vi "init.vi"() -> (0 "error out":errorcluster, 3 "Modules":T1)   [LabVIEW 2025]
uses:
  <vilib>/Utility/sysdir.llb/System Directory Type.ctl
  Libraries/USB IO/USB IO.lvlib
  Libraries/Power Supply/Power Supply.lvlib
  Libraries/Motor/Motor.lvlib
  Libraries/Wheatstone Bridge/Wheatstone Bridge.lvlib
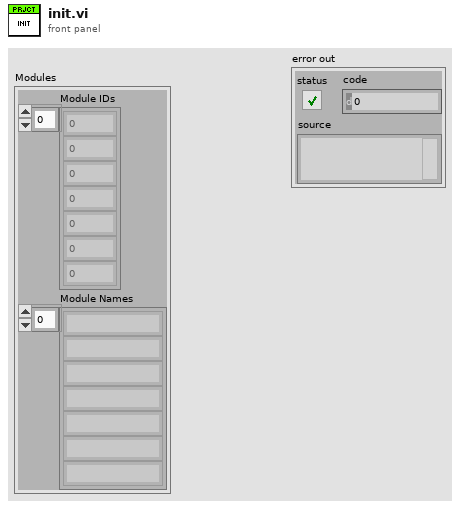
[diagram p1: front panel]
types:
  T1 = cluster{"Module IDs":i32[], "Module Names":string[]}
  T2 = typedef "System Directory Type.ctl" = i32
  T3 = typedef "Hardware Selection.ctl" = enum16{"Simulation", "USB-6000", "USB-6001", "Arduino Uno"}
  T4 = typedef "hardware-selection.ctl" = enum16{"Parent", "Simulation", "PSP-603"}
  T5 = typedef "Motor Selection.ctl" = enum16{"Stepper", "CL57RS"}
  T6 = typedef "Wheatstone Bridge.lvlib/Wheatstone Bridge.lvclass/Hardware Selection.ctl" = enum16{"Wheatstone Bridge", "NI-9237"}
  T7 = cluster{"IO":T3, "Power_supply":T4, "Motor":T5, "Torque Transducer":T6}
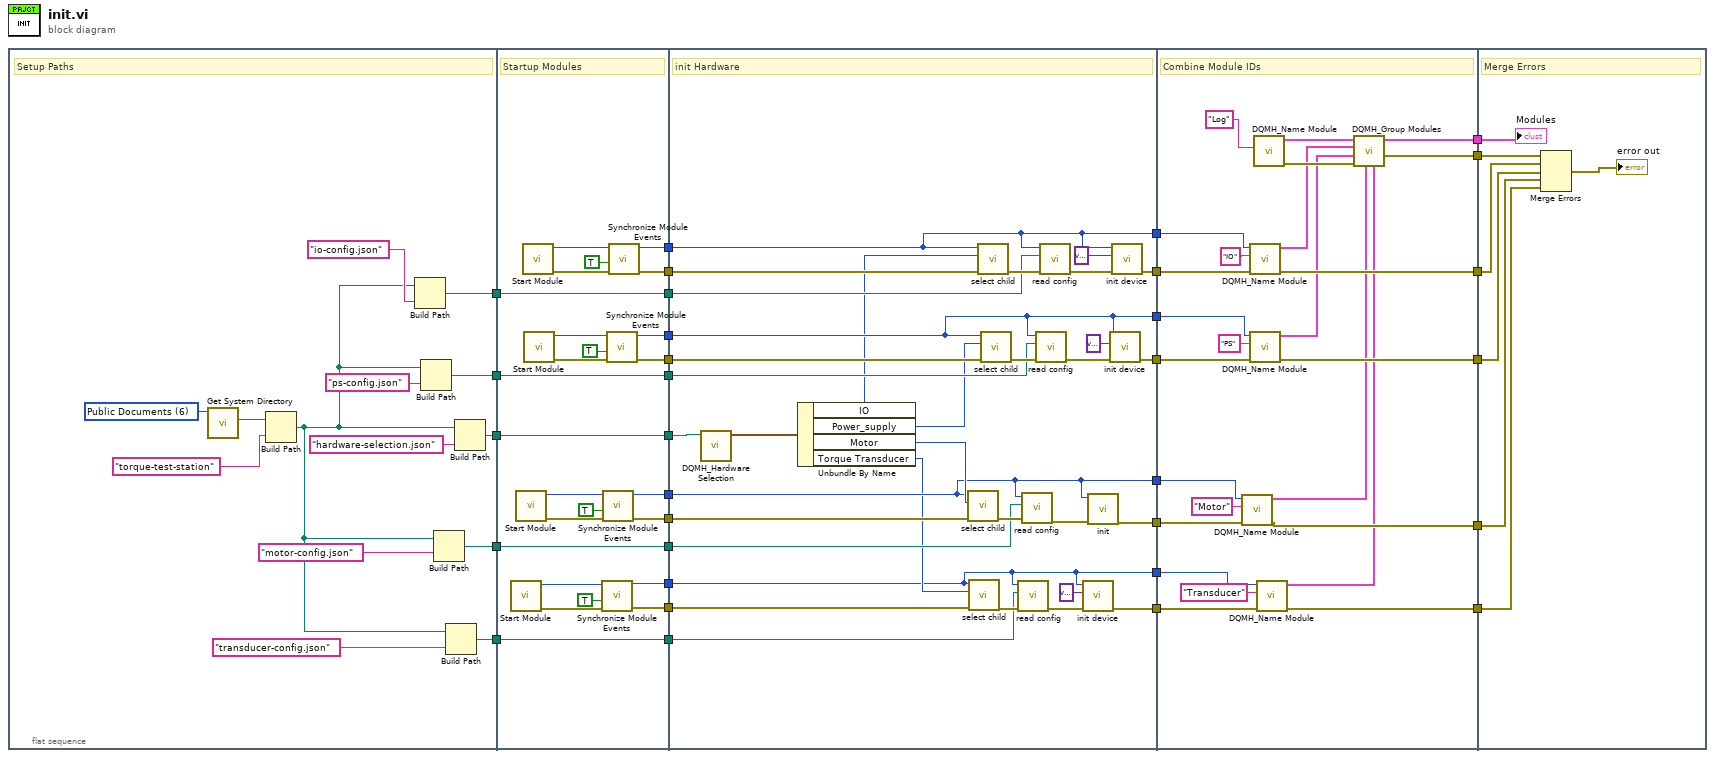
[diagram p0: block diagram]
diagram:
  n1 = flat-sequence {
    tunnel: [w42] -> w28
    tunnel: [w40] -> w22
    tunnel: [w38] -> w16
    tunnel: [w37] -> w8
    tunnel: [w33] -> w4
    tunnel: [w68] -> w30
    tunnel: [w67] -> w29
    tunnel: w28 -> [w66]
    tunnel: [w66] -> w27
    tunnel: [w62] -> w23
    tunnel: w22 -> [w62]
    tunnel: [w61] -> w21
    tunnel: [w60] -> w20
    tunnel: w16 -> [w59]
    tunnel: [w59] -> w15
    tunnel: [w55] -> w14
    tunnel: [w54] -> w13
    tunnel: [w53] -> w12
    tunnel: w8 -> [w53]
    tunnel: [w49] -> w7
    tunnel: [w48] -> w6
    tunnel: [w47] -> w5
    tunnel: w4 -> [w47]
    tunnel: w30 -> [w99]
    tunnel: w29 -> [w104]
    tunnel: w27 -> [w102]
    tunnel: [w99] -> w26
    tunnel: [w98] -> w25
    tunnel: w23 -> [w95]
    tunnel: w21 -> [w92]
    tunnel: w20 -> [w97]
    tunnel: [w92] -> w19
    tunnel: [w91] -> w18
    tunnel: w15 -> [w90]
    tunnel: w14 -> [w81]
    tunnel: w13 -> [w86]
    tunnel: w12 -> [w83]
    tunnel: [w81] -> w11
    tunnel: [w80] -> w10
    tunnel: w7 -> [w72]
    tunnel: w6 -> [w79]
    tunnel: w5 -> [w76]
    tunnel: [w73] -> w3
    tunnel: [w72] -> w2
    tunnel: [w126] -> w32
    tunnel: [w125] -> w31
    tunnel: w26 -> [w124]
    tunnel: w25 -> [w122]
    tunnel: [w120] -> w24
    tunnel: w19 -> [w119]
    tunnel: w18 -> [w118]
    tunnel: [w115] -> w17
    tunnel: w11 -> [w114]
    tunnel: w10 -> [w113]
    tunnel: [w110] -> w9
    tunnel: w3 -> [w109]
    tunnel: w2 -> [w108]
    tunnel: [w105] -> w1
    tunnel: w32 -> [w135]
    tunnel: w31 -> [w136]
    tunnel: w24 -> [w133]
    tunnel: w17 -> [w132]
    tunnel: w9 -> [w131]
    tunnel: w1 -> [w130]
    frame #0 {
      w46 = T2 6 items=["User Home"=0, "User Desktop"=1, "User Documents"=2, "User Application Data"=3, "User Preferences"=4, "User Temporary"=5, "Public Documents"=6, "Public Application Data"=7, "Public Preferences"=8, "Public Cache"=13, "System Core Libraries"=9, "System Installed Libraries"=10, "Application Files"=11, "Boot Volume Root"=12] ("system directory type")
      # "Setup Paths"
      n2 = call <vilib>:"Get System Directory.vi"("system directory type"=w46) -> ("system directory"=w45:path)  [unwired: 10 in]
      n3 = Build Path(base path=w45, name or relative path="torque-test-station") -> (appended path=w34:path)
      n4 = Build Path(base path=w34, name or relative path="io-config.json") -> (appended path=w42:path)
      n5 = Build Path(base path=w34, name or relative path="ps-config.json") -> (appended path=w40:path)
      n6 = Build Path(base path=w34, name or relative path="motor-config.json") -> (appended path=w37:path)
      n7 = Build Path(base path=w34, name or relative path="transducer-config.json") -> (appended path=w33:path)
      n8 = Build Path(base path=w34, name or relative path="hardware-selection.json") -> (appended path=w38:path)
    }
    frame #1 {
      # "Startup Modules"
      n9 = call "Start Module.vi"() -> ("error out"=w51:errorcluster, "Module ID"=w52:i32)  [unwired: 7 in, 3 out]
      n10 = call "Start Module.vi"() -> ("error out"=w57:errorcluster, "Module ID"=w58:i32)  [unwired: 7 in, 3 out]
      n11 = call "Start Module.vi"() -> ("error out"=w70:errorcluster, "Module ID"=w71:i32)  [unwired: 7 in, 3 out]
      n12 = call "Start Module.vi"() -> ("error out"=w64:errorcluster, "Module ID"=w65:i32)  [unwired: 7 in, 3 out]
      n13 = call "Synchronize Module Events.vi"("error in"=w51, "Wait for Event Sync?"=TRUE, "Module ID in"=w52) -> ("error out"=w48:errorcluster, "Module ID out"=w49:i32)  [unwired: 7 in]
      n14 = call "Synchronize Module Events.vi"("error in"=w57, "Wait for Event Sync?"=TRUE, "Module ID in"=w58) -> ("error out"=w54:errorcluster, "Module ID out"=w55:i32)  [unwired: 7 in]
      n15 = call "Synchronize Module Events.vi"("error in"=w64, "Wait for Event Sync?"=TRUE, "Module ID in"=w65) -> ("error out"=w60:errorcluster, "Module ID out"=w61:i32)  [unwired: 7 in]
      n16 = call "Synchronize Module Events.vi"("error in"=w70, "Wait for Event Sync?"=TRUE, "Module ID in"=w71) -> ("error out"=w67:errorcluster, "Module ID out"=w68:i32)  [unwired: 7 in]
    }
    frame #2 {
      # "init Hardware"
      n17 = call "DQMH_Hardware Selection.vi"("File Path"=w90) -> ("Data out"=w89:T7)  [unwired: 10 in]
      n18 = Unbundle By Name(w89) -> ("IO"=w88:T3, "Power_supply"=w87:T4, "Motor"=w85:T5, "Torque Transducer"=w78:T6)
      n19 = call "select child.vi"("error in"=w86, "Enum"=w85, "Module ID"=w81) -> ("error out"=w84:errorcluster)  [unwired: 7 in, 1 out]
      n20 = call "select child.vi"("error in"=w79, "Hardware Selection"=w78, "Module ID"=w72) -> ("error out"=w77:errorcluster)  [unwired: 7 in, 1 out]
      n21 = call "select child.vi"("error in"=w104, "Hardware"=w88, "Module ID"=w99) -> ("error out"=w103:errorcluster)  [unwired: 7 in, 1 out]
      n22 = call "select child.vi"("error in"=w97, "Enum"=w87, "Module ID"=w92) -> ("error out"=w96:errorcluster)  [unwired: 7 in, 1 out]
      n23 = call "read config.vi"("error in"=w77, "File Path"=w76, "Module ID"=w72) -> ("error out"=w75:errorcluster)  [unwired: 7 in, 1 out]
      n24 = call "read config.vi"("error in"=w84, "json file path"=w83, "Module ID"=w81) -> ("error out"=w82:errorcluster)  [unwired: 7 in, 1 out]
      n25 = call "read config.vi"("error in"=w96, "config json file"=w95, "Module ID"=w92) -> ("error out"=w94:errorcluster)  [unwired: 7 in, 1 out]
      n26 = call "read config.vi"("error in"=w103, "Path"=w102, "Module ID"=w99) -> ("error out"=w101:errorcluster)  [unwired: 7 in, 1 out]
      n27 = call "init device.vi"("error in"=w75, "Variant"=variant, "Module ID"=w72) -> ("error out"=w73:errorcluster)  [unwired: 7 in, 1 out]
      n28 = call "init.vi"("error in"=w82, "Module ID"=w81) -> ("error out"=w80:errorcluster)  [unwired: 8 in, 1 out]
      n29 = call "init device.vi"("error in"=w94, "Variant"=variant, "Module ID"=w92) -> ("error out"=w91:errorcluster)  [unwired: 7 in, 1 out]
      n30 = call "init device.vi"("error in"=w101, "Variant"=variant, "Module ID"=w99) -> ("error out"=w98:errorcluster)  [unwired: 7 in, 1 out]
    }
    frame #3 {
      # "Combine Module IDs"
      n31 = call "DQMH_Name Module.vi"("error in"=w113, "String"="Motor", "Module ID in"=w114) -> ("error out"=w110:errorcluster, "input cluster"=w111:T1)  [unwired: 7 in]
      n32 = call "DQMH_Name Module.vi"("error in"=w122, "String"="IO", "Module ID in"=w124) -> ("error out"=w120:errorcluster, "input cluster"=w121:T1)  [unwired: 7 in]
      n33 = call "DQMH_Name Module.vi"("error in"=w118, "String"="PS", "Module ID in"=w119) -> ("error out"=w115:errorcluster, "input cluster"=w116:T1)  [unwired: 7 in]
      n34 = call "DQMH_Name Module.vi"("String"="Log") -> ("error out"=w127:errorcluster, "input cluster"=w128:T1)  [unwired: 9 in]
      n35 = call "DQMH_Name Module.vi"("error in"=w109, "String"="Transducer", "Module ID in"=w108) -> ("error out"=w105:errorcluster, "input cluster"=w106:T1)  [unwired: 7 in]
      n36 = call "DQMH_Group Modules.vi"("Module 5"=w106, "Module 4"=w111, "error in (no error)"=w127, "Module 3"=w116, "Module 2"=w121, "Module 1"=w128) -> ("error out"=w126:errorcluster, "Modules"=w125:T1)  [unwired: 4 in]
    }
    frame #4 {
      # "Merge Errors"
      n37 = Merge Errors(w135, w133, w132, w131, w130) -> (→"error out":errorcluster)
      "Modules" <- w136
    }
  }
